vi "ModbusIODriver.vi"(8 "Motor Speed Controls":T1 {"SetSpeed 2" min=0.0; "SetSpeed1" min=0.0 max=360.0}, 9 "Motor Bool Control":T2, 10 "Write":bool, 11 "stop":bool) -> (0 "Motor Status Indicators":T3, 1 "Motor Bool Control Indicators":T4, 3 "Read Speed":T5 {"ReadSpeed2" format="%.2f"; "ReadSpeed1" format="%.2f"; "SetSpeed2" format="%.2f"; "SetSpeed1" format="%.2f"}, 5 "error IO":errorcluster)   [LabVIEW 2024]
uses:
  Torsjonsrigg/support/ReadSpeed.ctl
  Torsjonsrigg/support/MotorBoolControlsIndicators.ctl
  Torsjonsrigg/support/MotorStatusIndicators.ctl
  Torsjonsrigg/support/MotorBoolControls.ctl
  Torsjonsrigg/support/MotorSpeedControls.ctl
  <vilib>/Modbus/master/Modbus Master.lvclass
  <vilib>/Modbus/master/Create Master Instance (TCP).vi
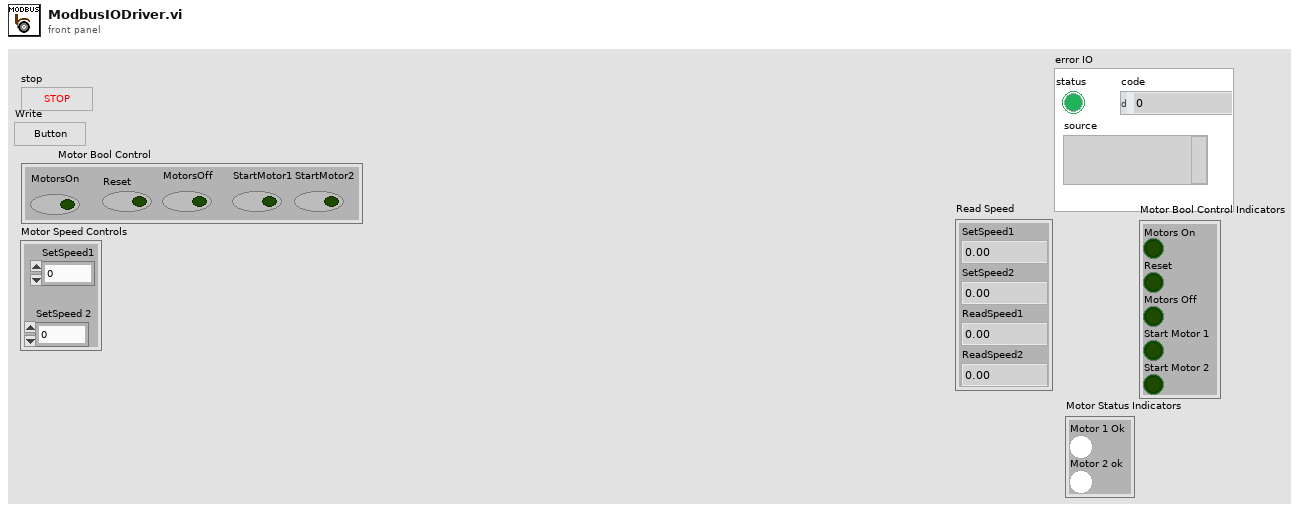
[diagram p1: front panel]
types:
  T1 = typedef "MotorSpeedControls.ctl" = cluster{"SetSpeed1":dbl, "SetSpeed 2":dbl}
  T2 = typedef "MotorBoolControls.ctl" = cluster{"MotorsOn":bool, "Reset":bool, "MotorsOff":bool, "StartMotor1":bool, "StartMotor2":bool}
  T3 = typedef "MotorStatusIndicators.ctl" = cluster{"Motor 1 Ok":bool, "Motor 2 ok":bool}
  T4 = typedef "MotorBoolControlsIndicators.ctl" = cluster{"Motors On":bool, "Reset":bool, "Motors Off":bool, "Start Motor 1 ":bool, "Start Motor 2":bool}
  T5 = typedef "ReadSpeed.ctl" = cluster{"SetSpeed1":dbl, "SetSpeed2":dbl, "ReadSpeed1":dbl, "ReadSpeed2":dbl}
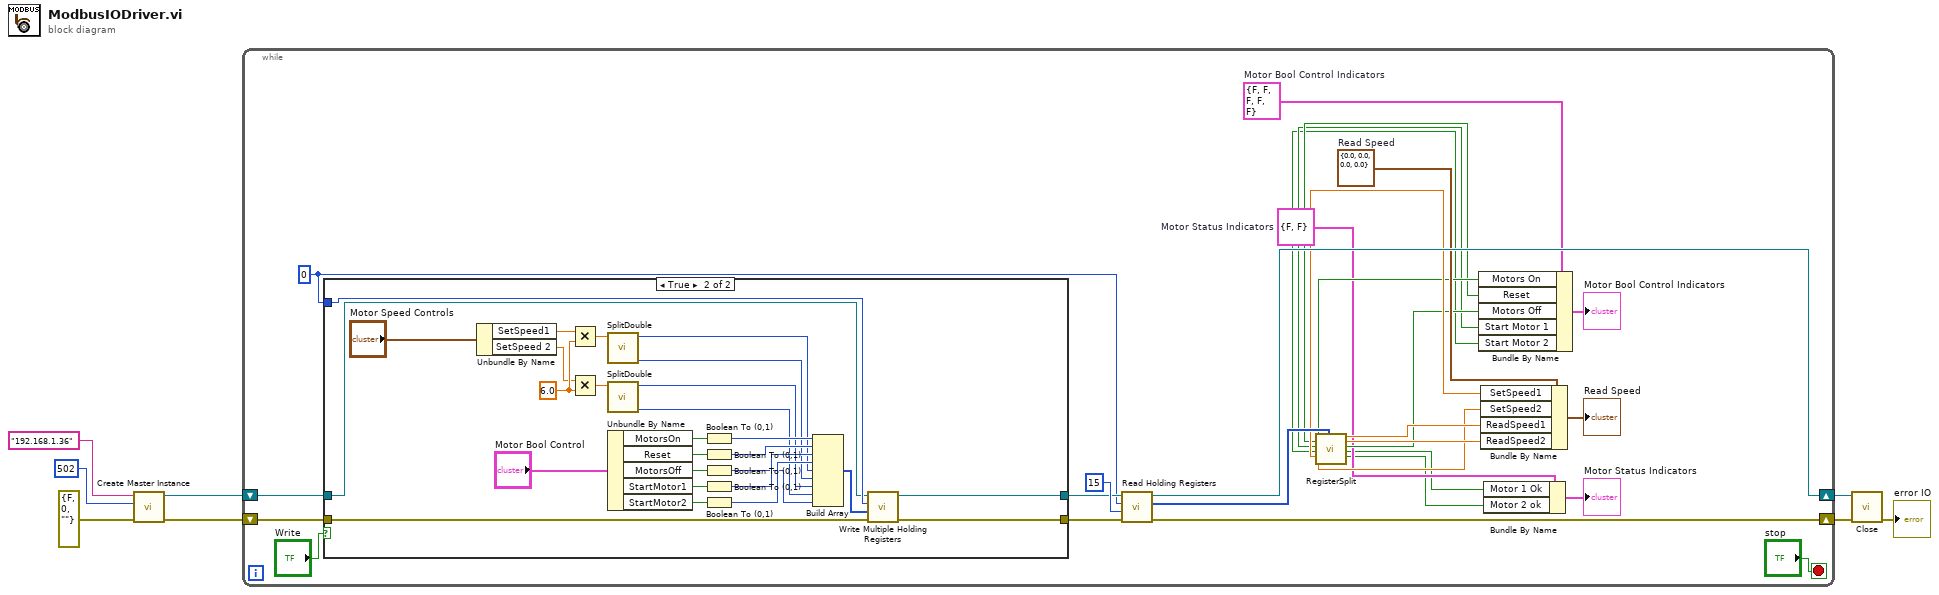
[diagram p0: block diagram]
diagram:
  n1 = call-poly <vilib>:"Create Master Instance.vi"("error in (no error)"=errorcluster {"status"=FALSE, "code"=0, "source"=""}, "port (502)"=u16 502, "address"="192.168.1.36") -> ("error out"=w4:errorcluster, "TCP master instance"=w5:refnum<class "Modbus Master.lvclass">)  [unwired: 7 in]
  n2 = while {
    shift-right: [w35] -> w3
    shift-left: w5 -> [w30]
    shift-right: [w34] -> w2
    shift-left: w4 -> [w27]
    stop <- "stop" stop-if-true
    w12 = T3 {"Motor 1 Ok"=FALSE, "Motor 2 ok"=FALSE}  # Motor Status Indicators
    w19 = T4 {"Motors On"=FALSE, "Reset"=FALSE, "Motors Off"=FALSE, "Start Motor 1 "=FALSE, "Start Motor 2"=FALSE}  # Motor Bool Control Indicators
    w25 = T5 {"SetSpeed1"=0.0, "SetSpeed2"=0.0, "ReadSpeed1"=0.0, "ReadSpeed2"=0.0}  # Read Speed
    w26 = u16 0 ("starting address")
    n3 = case shown="True" "Write" {
      tunnel: w30 -> [w38 w39]
      tunnel: [w38 w65] -> w29
      tunnel: [w37 w64] -> w28
      tunnel: w27 -> [w37 w63]
      tunnel: w26 -> [_ w62]
      frame False {
      }
      frame True {
        w51 = 6.0 ("y")
        n4 = Unbundle By Name("Motor Speed Controls") -> ("SetSpeed1"=w49:dbl, "SetSpeed 2"=w48:dbl)
        n5 = Multiply(x=w49, y=w51) -> (x*y=w53:dbl)
        n6 = Multiply(x=w48, y=w51) -> (x*y=w52:dbl)
        n7 = call "SplitDouble.vi"("number"=w53) -> ("Low"=w44:i16, "High"=w45:i16)  [unwired: 9 in]
        n8 = call "SplitDouble.vi"("number"=w52) -> ("Low"=w42:i16, "High"=w43:i16)  [unwired: 9 in]
        n9 = Unbundle By Name("Motor Bool Control") -> ("MotorsOn"=w61:bool, "Reset"=w59:bool, "MotorsOff"=w58:bool, "StartMotor1"=w57:bool, "StartMotor2"=w56:bool)
        n10 = Boolean To (0,1)(Boolean=w61) -> (0, 1=w55:i16)
        n11 = Boolean To (0,1)(Boolean=w59) -> (0, 1=w54:i16)
        n12 = Boolean To (0,1)(Boolean=w58) -> (0, 1=w41:i16)
        n13 = Boolean To (0,1)(Boolean=w57) -> (0, 1=w47:i16)
        n14 = Boolean To (0,1)(Boolean=w56) -> (0, 1=w46:i16)
        n15 = Build Array(w55, w54, w47, w46, w45, w44, w43, w42, w41) -> (w40:i16[])
        n16 = call-dynamic "Write Multiple Holding Registers.vi"("error in (no error)"=w63, "holding register values"=w40, "starting address"=w62, "Modbus master in"=w39) -> ("error out"=w64:errorcluster, "Modbus master out"=w65:refnum<class "Modbus Master.lvclass">)  [unwired: 6 in]
      }
    }
    n17 = call-dynamic "Read Holding Registers.vi"("error in (no error)"=w28, "number of holding registers"=u16 15, "starting address"=w26, "Modbus master in"=w29) -> ("error out"=w34:errorcluster, "register values"=w33:u16[], "Modbus master out"=w35:refnum<class "Modbus Master.lvclass">)  [unwired: 5 in]
    n18 = call "RegisterSplit.vi"("register values"=w33) -> ("[0] Motor1On"=w16:bool, "[1]Motor2On"=w15:bool, "[2]StartMotor1"=w14:bool, "[3]StartMotor2"=w13:bool, "[4] SetSpeed1"=w21:dbl, "[5] SetSpeed2"=w20:dbl, "[7]ReadSpeed1"=w23:dbl, "[8] ReadSpeed2"=w22:dbl, "[6] MotorsOff"=w17:bool, "[9]Motor1Ok"=w10:bool, "[10]Motor2Ok"=w9:bool)  [unwired: 8 in]
    n19 = Bundle By Name(cluster=w19, "Motors On"=w16, "Reset"=w15, "Motors Off"=w17, "Start Motor 1"=w14, "Start Motor 2"=w13) -> (→"Motor Bool Control Indicators":T4)
    n20 = Bundle By Name(cluster=w25, "SetSpeed1"=w21, "SetSpeed2"=w20, "ReadSpeed1"=w23, "ReadSpeed2"=w22) -> (→"Read Speed":T5)
    n21 = Bundle By Name(cluster=w12, "Motor 1 Ok"=w10, "Motor 2 ok"=w9) -> (→"Motor Status Indicators":T3)
  }
  n22 = call-dynamic "Close.vi"("error in (no error)"=w2, "Modbus master in"=w3) -> ("error out"=→"error IO":errorcluster)  [unwired: 9 in]
